vi "Set List Options.vi"(8 "error in (no error)":errorcluster, 10 "Drop-down List Options":string[](array[string]), 11 "List Data Type in":refnum<class "List Data Type.lvclass">) -> (0 "error out":errorcluster, 3 "List Data Type out":refnum<class "List Data Type.lvclass">)   [LabVIEW 2018, in "List Data Type.lvclass"]
uses:
  List Data Type.lvclass
  List Data Type.lvclass/List Data Type.ctl
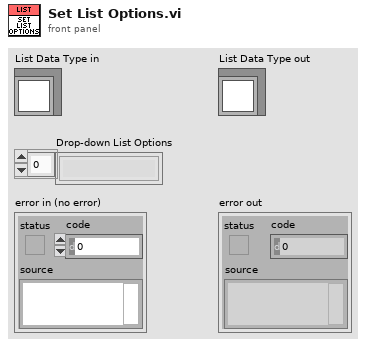
[diagram p1: front panel]
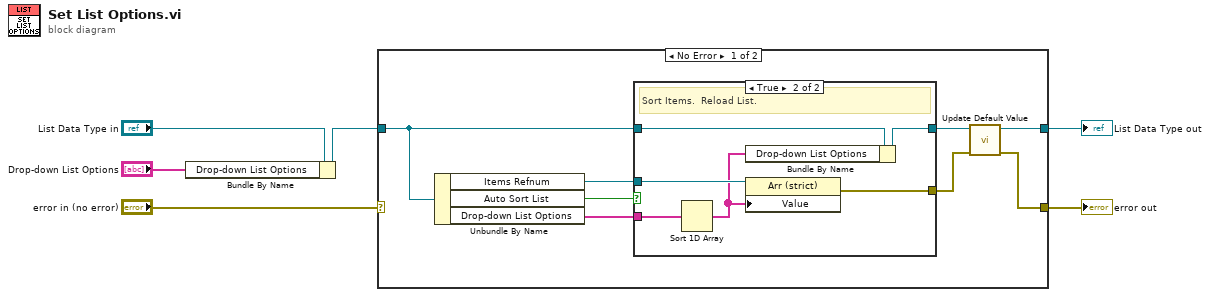
[diagram p0: block diagram]
diagram:
  n1 = Bundle By Name(cluster="List Data Type in", "Drop-down List Options"="Drop-down List Options") -> (w2:refnum<class "List Data Type.lvclass">)
  n2 = case shown="No Error" "error in (no error)" {
    selector: "error in (no error)" -> [_ w23]
    tunnel: [w8 w23] -> w5
    tunnel: [w10 w22] -> w4
    tunnel: w2 -> [w11 w22]
    frame No Error {
      n3 = Unbundle By Name(w11) -> ("Items Refnum"=w12:refnum<vi>, "Auto Sort List"=w14:bool, "Drop-down List Options"=w13:string[])
      n4 = case shown="True" w14 {
        tunnel: w13 -> [_ w21]
        tunnel: w12 -> [_ w20]
        tunnel: [_ w19] -> w7
        tunnel: w11 -> [w15 w18]
        tunnel: [w15 w16] -> w9
        frame False {
          # "Leave List Alone"
        }
        frame True {
          # "Sort Items.  Reload List."
          n5 = Sort 1D Array(array=w21) -> (sorted array=w17:string[])
          n6 = Bundle By Name(cluster=w18, "Drop-down List Options"=w17) -> (w16:refnum<class "List Data Type.lvclass">)
          n7 = property class="Arr (strict)"(reference=w20, "Value"=w17) -> (error out=w19:errorcluster)  [unwired: 1 in, 1 out]
        }
      }
      n8 = call "Update Default Value.vi"("error in (no error)"=w7, "List Data Type in"=w9) -> ("error out"=w8:errorcluster, "List Data Type out"=w10:refnum<class "List Data Type.lvclass">)  [unwired: 8 in]
    }
    frame Error {
    }
  }
  "error out" <- w5
  "List Data Type out" <- w4
